vi "test Acyclic Loopback with SDI.vi"(8 "error in":errorcluster, 11 "TestCase in":refnum<class "Single Board Loopback.lvclass">) -> (0 "error out":errorcluster, 3 "TestCase out":refnum<class "Single Board Loopback.lvclass">)   [LabVIEW 2024, in "Single Board Loopback.lvclass"]
uses:
  Single Board Loopback.lvclass
  C:/Program Files/National Instruments/LabVIEW 2024/vi.lib/NI/VeriStand Custom Device Testing Tools/VeriStandTestCase/VeriStandTestCase.lvclass
  <vilib>/numeric/Random Number (Range) U64.vi
  <vilib>/numeric/sub_Random U32.vi
  <vilib>/NI VeriStand/Execution/Workspace/NI VeriStand - Set Single Channel Value.vi
  <vilib>/addons/_JKI Toolkits/VI Tester/TestCase.llb/TestCase.lvclass
  <vilib>/NI VeriStand/Execution/Workspace/NI_VS Workspace ExecutionAPI.lvlib
  <vilib>/NI/VeriStand Custom Device Testing Tools/VeriStandTestUtilities/VeriStandTestUtilities.lvlib
  C:/Program Files/National Instruments/LabVIEW 2024/vi.lib/addons/_JKI Toolkits/VI Tester/TestCase.llb/TestCase.lvclass
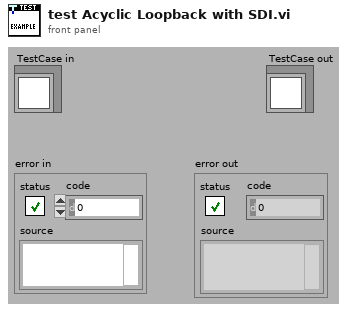
[diagram p1: front panel]
types:
  T1 = typedef "NI_VS Workspace ExecutionAPI.lvlib/WorkspaceAPI.ctl" = refnum<k24>
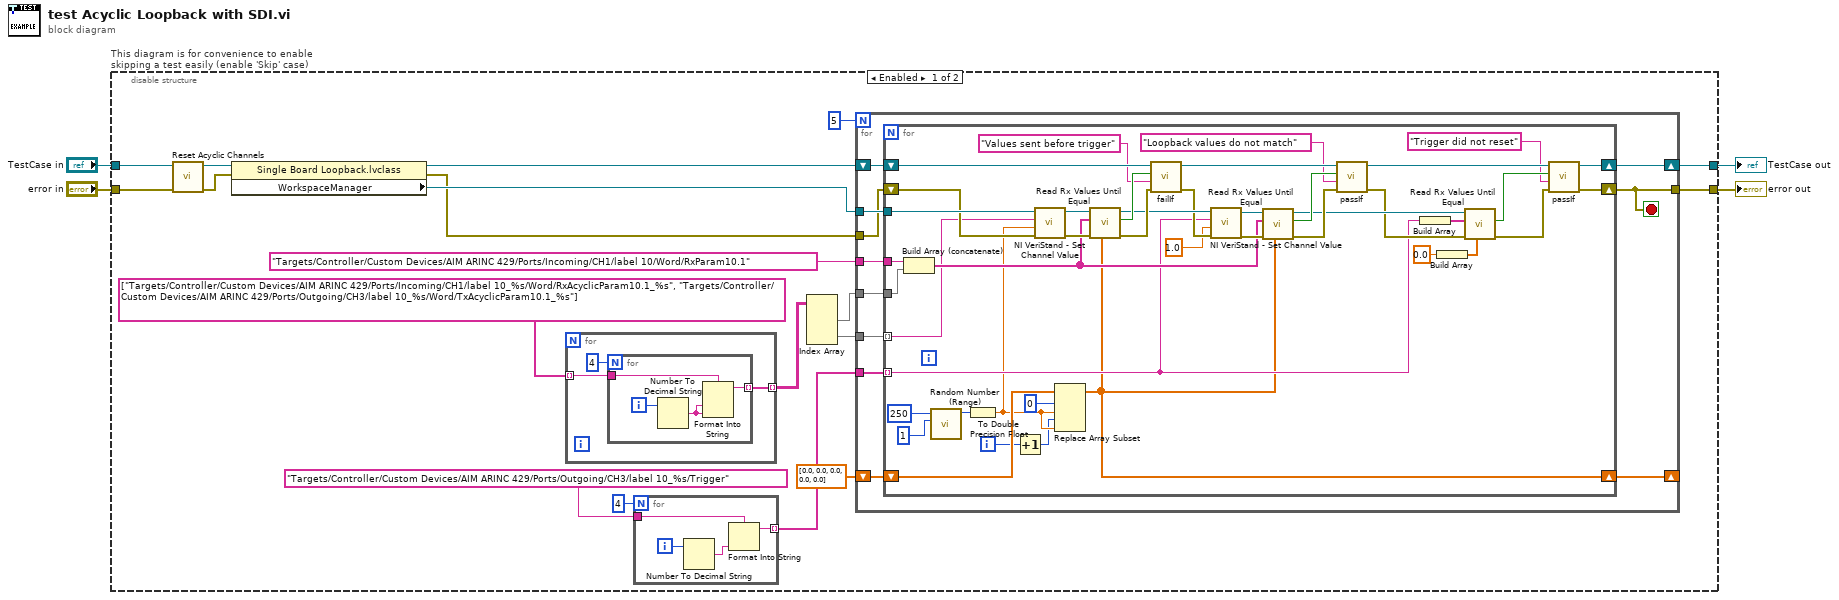
[diagram p0: block diagram]
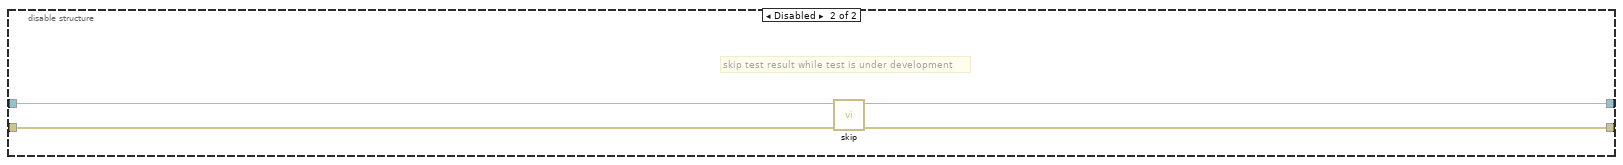
[diagram p2: hidden frame]
diagram:
  n1 = disable-structure "This diagram is for convenience to enable skipping a test easily (enable 'Skip' case)" shown="Enabled" {
    disable-tunnel: "TestCase in" -> [w14 w91]
    disable-tunnel: [w18 w89] -> w1
    disable-tunnel: [w17 w90] -> w3
    disable-tunnel: "error in" -> [w19 w88]
    frame Enabled {
      n2 = call "Reset Acyclic Channels.vi"("error in (no error)"=w19, "Single Board Loopback in"=w14) -> ("error out"=w15:errorcluster, "Single Board Loopback out"=w13:refnum<class "Single Board Loopback.lvclass">)  [unwired: 8 in]
      n3 = property class="Single Board Loopback.lvclass"(reference=w13, error in=w15) -> (reference out=w21:refnum<class "Single Board Loopback.lvclass">, error out=w22:errorcluster, "WorkspaceManager"=w23:T1)
      n4 = for {
        tunnel: [w30] -> w9 mode=indexing
        tunnel: string[] ["Targets/Controller/Custom Devices/AIM ARINC 429/Ports/Incoming/CH1/label 10_%s/Word/RxAcyclicParam10.1_%s", "Targets/Controller/Custom Devices/AIM ARINC 429/Ports/Outgoing/CH3/label 10_%s/Word/TxAcyclicParam10.1_%s"] -> [w29] mode=indexing
        n5 = for {
          N: 4 -> [_]
          tunnel: w29 -> [w31]
          tunnel: [w33] -> w30 mode=indexing
          i -> [w34]
          n6 = Number To Decimal String(number=w34) -> (decimal integer string=w32:string)  [unwired: 1 in]
          n7 = Format Into String(format string=w31, w32, w32) -> (resulting string=w33:string)  [unwired: 2 in, 1 out]
        }
      }
      n8 = for {
        N: 4 -> [_]
        tunnel: [w26] -> w6 mode=indexing
        tunnel: "Targets/Controller/Custom Devices/AIM ARINC 429/Ports/Outgoing/CH3/label 10_%s/Trigger" -> [w24]
        i -> [w27]
        n9 = Number To Decimal String(number=w27) -> (decimal integer string=w25:string)  [unwired: 1 in]
        n10 = Format Into String(format string=w24, w25) -> (resulting string=w26:string)  [unwired: 2 in, 1 out]
      }
      n11 = Index Array(array=w9) -> (element #1=w11:string[], element #2=w10:string[])  [unwired: 4 in]
      n12 = for {
        N: 5 -> [_]
        tunnel: w23 -> [w45]
        tunnel: w22 -> [w43]
        shift-right: [w41] -> w18
        shift-left: w21 -> [w44]
        tunnel: [w42] -> w17
        tunnel: "Targets/Controller/Custom Devices/AIM ARINC 429/Ports/Incoming/CH1/label 10/Word/RxParam10.1" -> [w40]
        tunnel: w10 -> [w39]
        tunnel: w6 -> [w38]
        tunnel: w11 -> [w37]
        shift-right: [w36] -> _
        shift-left: dbl[] [0.0, 0.0, 0.0, 0.0, 0.0] -> [w35]
        stop <- w42 stop-if-true
        n13 = for {
          tunnel: w45 -> [w86]
          tunnel: w40 -> [w61]
          shift-right: [w70] -> w41
          shift-left: w44 -> [w82]
          shift-right: [w72] -> w42
          shift-left: w43 -> [w80]
          tunnel: w39 -> [w57] mode=indexing
          tunnel: w38 -> [w56] mode=indexing
          tunnel: w37 -> [w52]
          shift-right: [w49] -> w36
          shift-left: w35 -> [w51]
          i -> [w48]
          n14 = Build Array (concatenate)(w61, w52) -> (w58:string[])
          n15 = call-poly <vilib>:"Random Number (Range).vi"("lower bound (0)"=u64 1 ("upper bound (100)"), "upper bound (100)"=u64 250) -> ("number"=w62:u64)  [unwired: 9 in]
          n16 = To Double Precision Float(number=w62) -> (double precision float=w47:dbl)
          n17 = Increment(x=w48) -> (x+1=w46:i32)
          n18 = call-poly <vilib>:"NI VeriStand - Set Channel Value.vi"("error in (no error)"=w80, "Value"=w47, "Channel"=w57, "WorkspaceManager in"=w86) -> ("error out"=w83:errorcluster, "WorkspaceManager out"=w85:T1)  [unwired: 6 in]
          n19 = Replace Array Subset(array=w51, new element #1=w47, index #1=0 ("index"), new element #2=w47, index #2=w46) -> (w49:dbl[])
          n20 = call <vilib>:"Read Rx Values Until Equal.vi"("expected values"=w49, "error in"=w83, "Rx aliases"=w58, "workspace manager in"=w85) -> ("error out"=w84:errorcluster, "values equal expected"=w81:bool, "workspace manager out"=w79:T1)  [unwired: 5 in]
          n21 = call-dynamic "failIf.vi"("error in (no error)"=w84, "message (\"\")"="Values sent before trigger" ("message (\"\")"), "fail"=w81, "TestCase in"=w82) -> ("error out"=w78:errorcluster, "TestCase out"=w73:refnum<class "Single Board Loopback.lvclass">)  [unwired: 6 in]
          n22 = call-poly <vilib>:"NI VeriStand - Set Channel Value.vi"("error in (no error)"=w78, "Value"=1.0, "Channel"=w56, "WorkspaceManager in"=w79) -> ("error out"=w76:errorcluster, "WorkspaceManager out"=w77:T1)  [unwired: 6 in]
          n23 = call <vilib>:"Read Rx Values Until Equal.vi"("expected values"=w49, "error in"=w76, "Rx aliases"=w58, "workspace manager in"=w77) -> ("error out"=w74:errorcluster, "values equal expected"=w75:bool, "workspace manager out"=w68:T1)  [unwired: 5 in]
          n24 = call-dynamic "passIf.vi"("error in (no error)"=w74, "message (\"\")"="Loopback values do not match" ("message (\"\")"), "pass"=w75, "TestCase in"=w73) -> ("error out"=w67:errorcluster, "TestCase out"=w71:refnum<class "Single Board Loopback.lvclass">)  [unwired: 6 in]
          n25 = Build Array(w56) -> (w55:string[])
          n26 = Build Array(0.0) -> (w53:dbl[])
          n27 = call <vilib>:"Read Rx Values Until Equal.vi"("expected values"=w53, "error in"=w67, "Rx aliases"=w55, "workspace manager in"=w68) -> ("error out"=w66:errorcluster, "values equal expected"=w69:bool)  [unwired: 5 in, 1 out]
          n28 = call-dynamic "passIf.vi"("error in (no error)"=w66, "message (\"\")"="Trigger did not reset" ("message (\"\")"), "pass"=w69, "TestCase in"=w71) -> ("error out"=w72:errorcluster, "TestCase out"=w70:refnum<class "Single Board Loopback.lvclass">)  [unwired: 6 in]
        }
      }
    }
    frame Disabled {
      # "skip test result while test is under development"
      n29 = call <vilib>:"skip.vi"("error in (no error)"=w88, "TestCase in"=w91) -> ("error out"=w90:errorcluster, "TestCase out"=w89:refnum<class "Single Board Loopback.lvclass">)  [unwired: 8 in]
    }
  }
  "error out" <- w3
  "TestCase out" <- w1
